vi "DBC Sync Value To CANFD Msg.vi"(9 "pCANFDMsg":u32, 10 "pMsgName":string, 11 "DBCHandle":cluster{}) -> (1 "pCANFDMsg out":u32, 2 "pMsgName out":string, 3 "function return":i32)   [LabVIEW 2010, in "dbc_parser.lvlib"]
doc: "int WINAPI DBC_SyncValueToCANFDMsg(long long DBCHandle, char* pMsgName, void* pCANFDMsg);"
uses:
  dbc_parser.lvlib
  USB2XXX/trunk/USB2XXX/USB2XXX/vs2019/Release/USB2XXX.dll
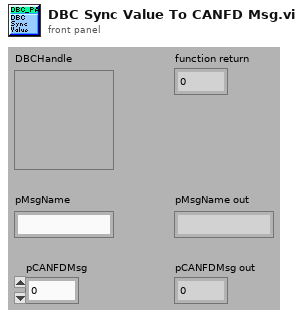
[diagram p1: front panel]
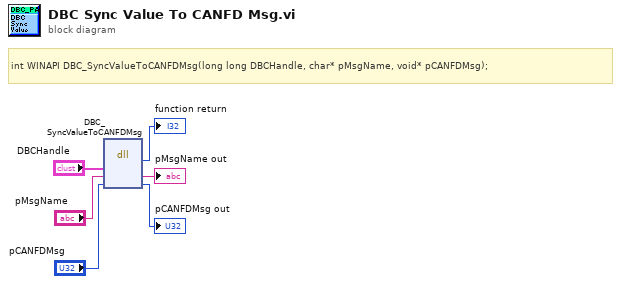
[diagram p0: block diagram]
diagram:
  # "int WINAPI DBC_SyncValueToCANFDMsg(long long DBCHandle, char* pMsgName, void* pCANFDMsg);"
  n1 = dll-call lib="E:/Projects/USB2XXX/trunk/USB2XXX/USB2XXX/vs2019/Release/USB2XXX.*" fn="DBC_SyncValueToCANFDMsg"("DBCHandle"="DBCHandle", "pMsgName"="pMsgName", "pCANFDMsg"="pCANFDMsg") -> (→"function return":i32, "pMsgName"=→"pMsgName out":string, "pCANFDMsg"=→"pCANFDMsg out":u32)  [unwired: 4 in, 2 out]
